vi "删除启动项.vi"(8 "error in (no error)":errorcluster caption="错误输入（无错误）", 11 "启动文件路径":path) -> (0 "error out":errorcluster caption="错误输出", 3 "删除标记":bool)   [LabVIEW 2016]
uses:
  <vilib>/registry/registry.llb/Registry RtKey.ctl
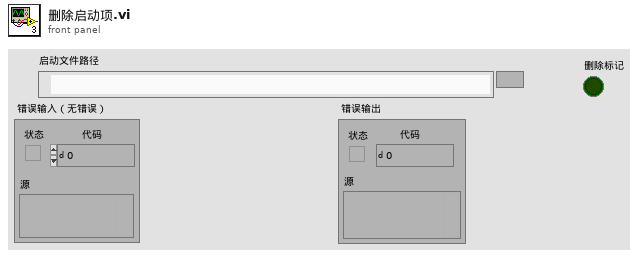
[diagram p1: front panel]
types:
  T1 = typedef "Registry RtKey.ctl" = enum32{"HKEY_CLASSES_ROOT", "HKEY_CURRENT_USER", "HKEY_LOCAL_MACHINE", "HKEY_USERS", "HKEY_PERFORMANCE_DATA", "HKEY_CURRENT_CONFIG", "HKEY_DYN_DATA"}
  T2 = typedef "Registry refnum.ctl" = refnum<k1>
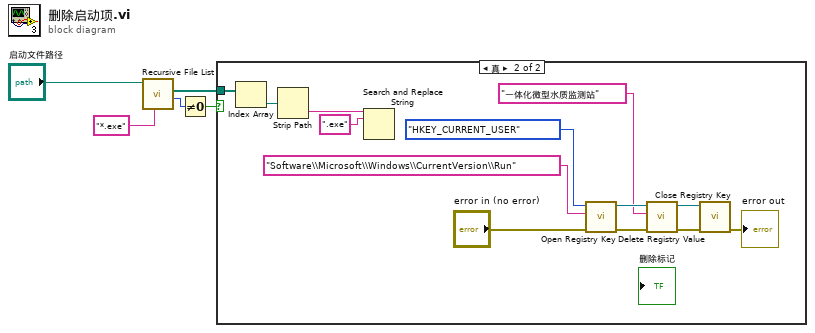
[diagram p0: block diagram]
diagram:
  n1 = call <vilib>:"Recursive File List.vi"("pattern"="*.exe", "Folder Path"="启动文件路径") -> ("Number of Files"=w2:i32, "All Files in Dir"=w3:path[])  [unwired: 5 in, 3 out]
  n2 = Not Equal To 0?(x=w2) -> (x != 0?=w1:bool)
  n3 = case shown="真" w1 {
    tunnel: w3 -> [_ w18]
    frame False {
    }
    frame True {
      n4 = Index Array(array=w18) -> (element=w17:path)  [unwired: 1 in]
      n5 = Strip Path(path=w17) -> (name=w16:string)  [unwired: 1 out]
      n6 = Search and Replace String(input string=w16, search string=".exe" ("搜索字符串")) -> ()  [unwired: 6 in, 4 out]
      n7 = call <vilib>:"Open Registry Key.vi"("error in (no error)"="error in (no error)", "subkey"="Software\\Microsoft\\Windows\\CurrentVersion\\Run", "root key (HKEY_LOCAL_MACHINE)"=Registry_RtKey."HKEY_CURRENT_USER") -> ("error out"=w10:errorcluster, "refnum out"=w12:T2)  [unwired: 7 in]
      n8 = call <vilib>:"Delete Registry Value.vi"("error in (no error)"=w10, "value"="一体化微型水质监测站", "refnum"=w12) -> ("error out"=w9:errorcluster, "refnum out"=w11:T2)  [unwired: 7 in]
      n9 = call <vilib>:"Close Registry Key.vi"("error in (no error)"=w9, "refnum"=w11) -> ("error out"=→"error out":errorcluster)  [unwired: 5 in]
    }
  }
